vi "Port Contains Mouse.vi"(0 "FSM.Node":refnum<class "FSM.Node.lvclass">, 7 "Coords":T1) -> (8 "contains mouse":bool, 10 "Location":cluster{"x":i16, "y":i16})   [LabVIEW 2020, in "FSM.Node.lvclass"]
uses:
  FSM.Node.lvclass
  <vilib>/Utility/miscctls.llb/LVPoint32TypeDef.ctl
  FSM.Node.lvclass/FSM.Node.ctl
  FSM.Port/FSM.Port.lvclass/FSM.Port.ctl
  FSM.Port/Read Location.vi
  FSM.Port/FSM.Port.lvclass
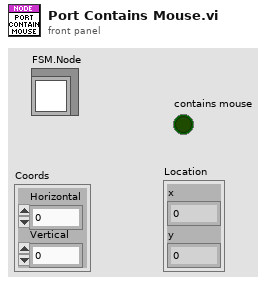
[diagram p1: front panel]
types:
  T1 = typedef "LVPoint32TypeDef.ctl" = cluster{"Horizontal":i32, "Vertical":i32}
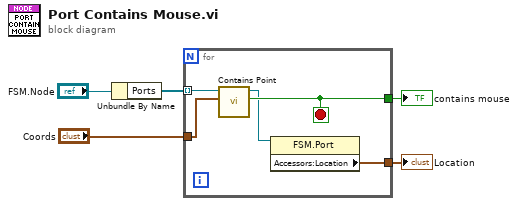
[diagram p0: block diagram]
diagram:
  n1 = Unbundle By Name("FSM.Node") -> ("Ports"=w4:refnum<class "FSM.Port.lvclass">[])
  n2 = for {
    tunnel: w4 -> [w10] mode=indexing
    tunnel: "Coords" -> [w9]
    tunnel: [w8] -> w2
    tunnel: [w6] -> w1
    stop <- w8 stop-if-true
    n3 = call "Contains Point.vi"("point"=w9, "Port in"=w10) -> ("contains point"=w8:bool, "Port out"=w7:refnum<class "FSM.Port.lvclass">)  [unwired: 7 in, 1 out]
    n4 = property class="FSM.Port"(reference=w7) -> ("Accessors:Location"=w6:cluster{"x":i16, "y":i16})  [unwired: 1 in, 2 out]
  }
  "contains mouse" <- w2
  "Location" <- w1
